vi "TrackAndRotateOmegaCopy.vi"() -> ()   [LabVIEW 2017]
doc: "This example shows how to monitor the measured value and how to set the position while open or closed loop controlled."
uses:
  <vilib>/ULx/Read.llb/ULx Read (Analog 2D DBL NChan NSamp).vi
panel:
  out "i":i32
  in  "Tab Control":enum32{"Page 1", "Page 2", "Page 3"}(tab)
  out "Connected":bool
  out "VISA resource name":refnum<visa-resource-name>="ASRL7::INSTR"
  out "Current position":dbl
  in  "Step size (deg.)":dbl=10.0
  in  "Abort 2":bool
  in  "Nb of steps":i32=50000
  out "Is Ready?":bool
  out "Times":dbl[](array[numeric])
  # "3"
  # "(c) 2012 piezosystem jena GmbH. ALL RIGHTS RESERVED."
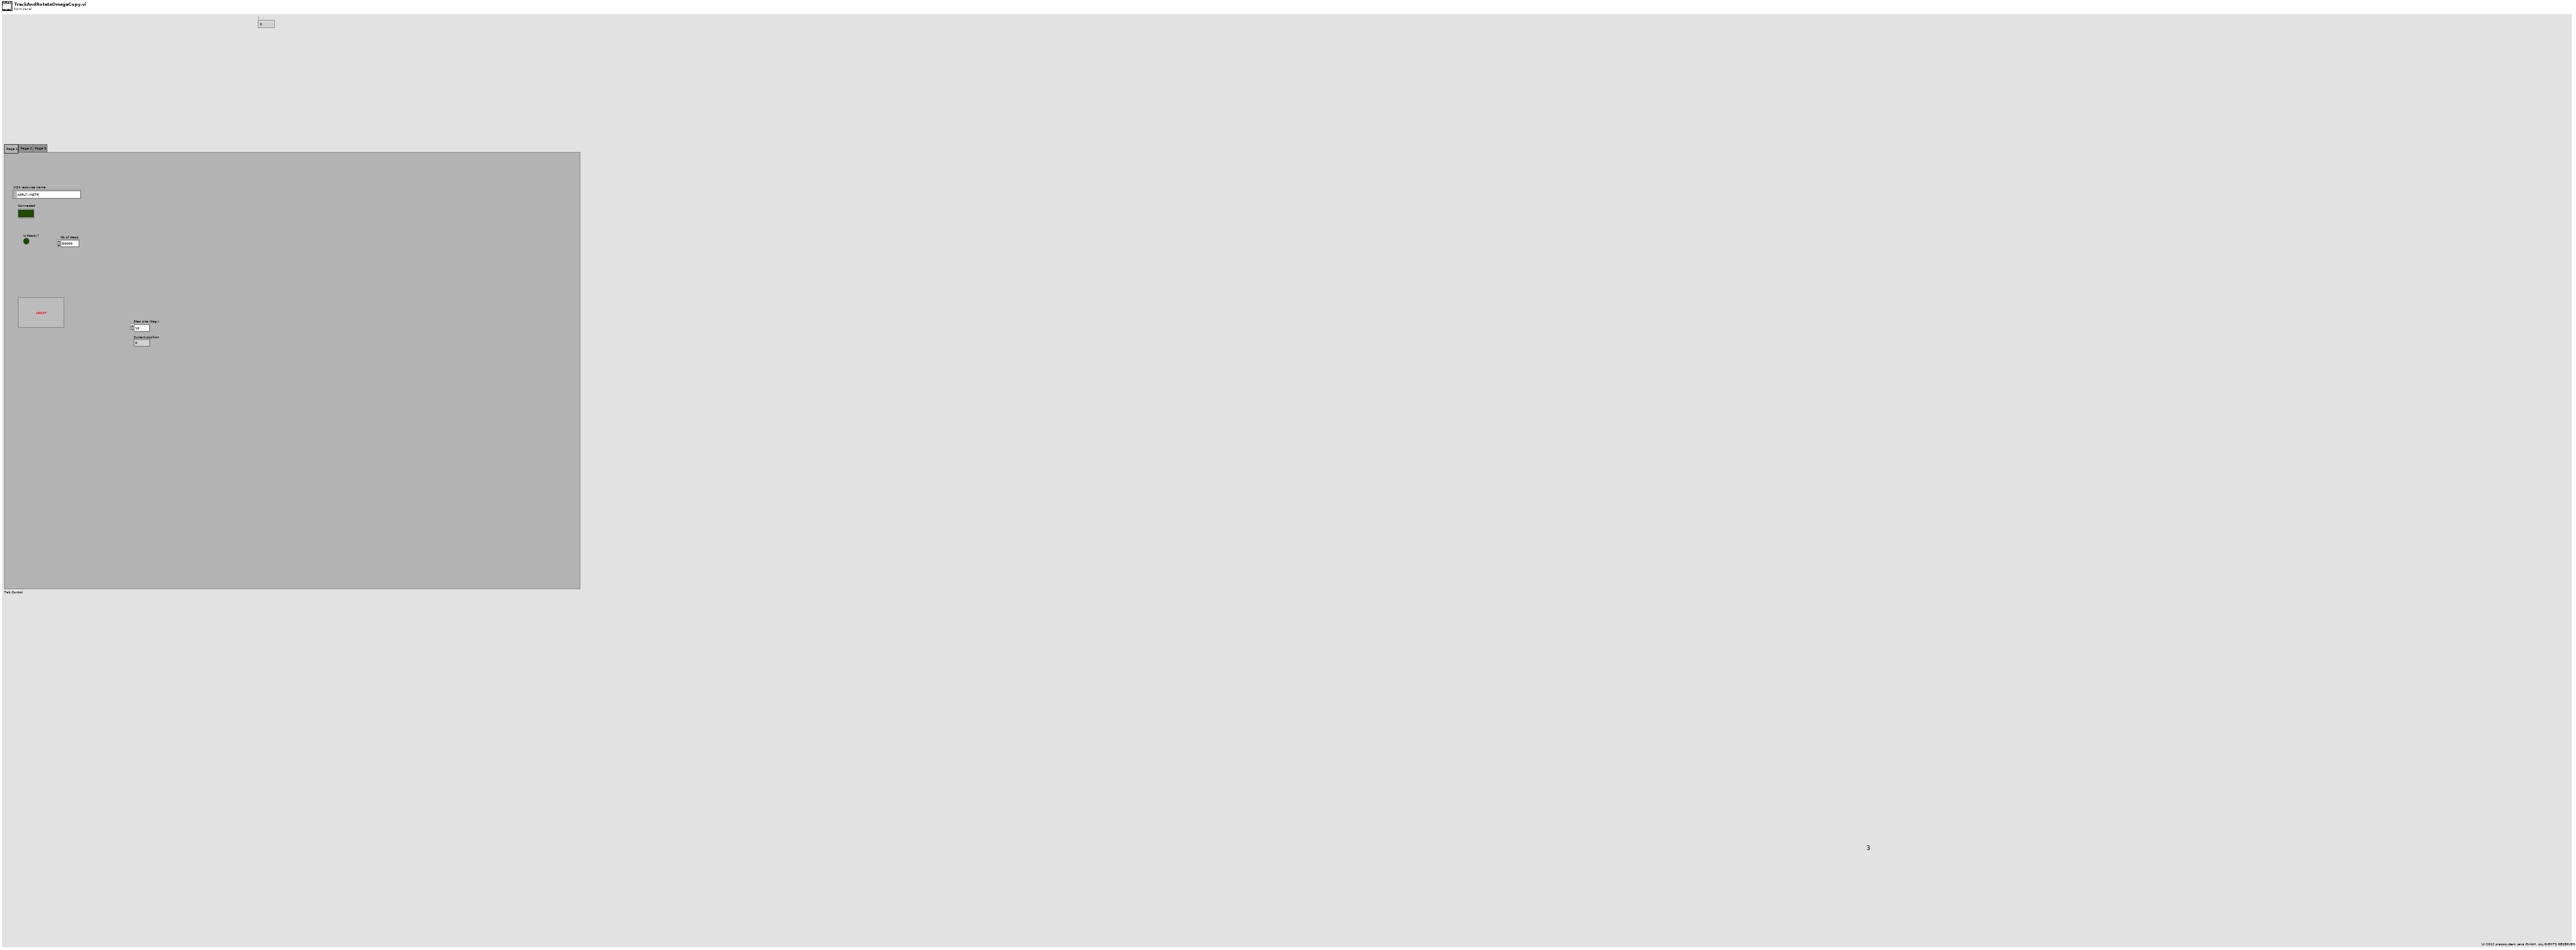
[diagram p1: front panel]
types:
  T1 = cluster{"VISA resource name":refnum<visa-resource-name>, "Device name":string, "Controller address":i32, "error":errorcluster}
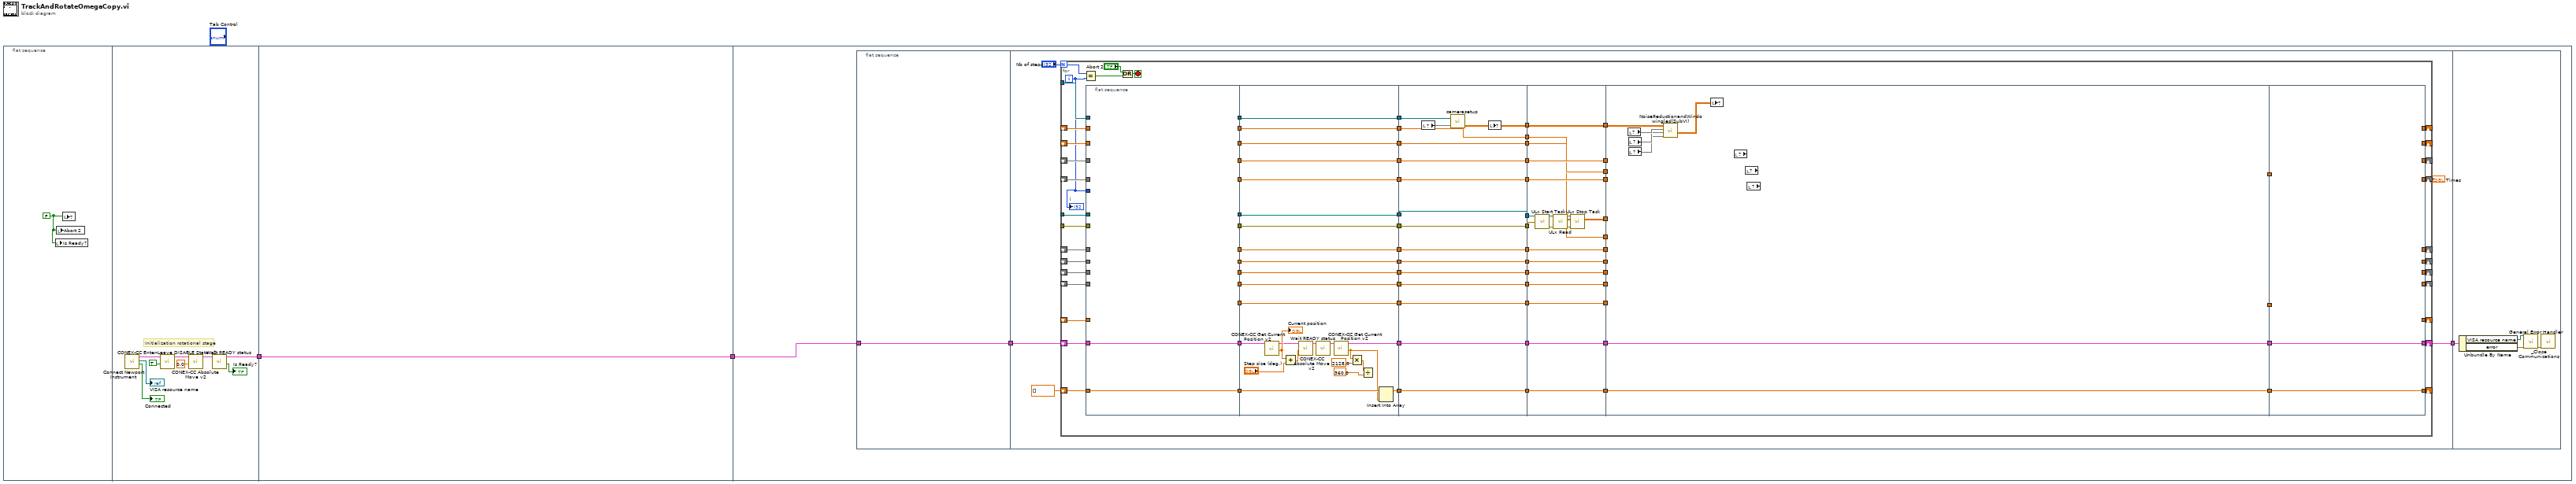
[diagram p0: block diagram]
diagram:
  n1 = flat-sequence {
    tunnel: [w7] -> w1
    tunnel: [w13] -> w2
    tunnel: w1 -> [w13]
    tunnel: w2 -> [w14]
    frame #0 {
      w3 = FALSE
      n2 = local write "Is Ready?"(w3) -> ()
      n3 = local write "Abort 2"(w3) -> ()
      n4 = local write item#-1(w3) -> ()
    }
    frame #1 {
      # "Initialization rotational stage"
      n5 = call <userlib>:"Connect Newport Instrument.vi"() -> ("Connected"=→"Connected":bool, "VISA resource name (duplicate)"=→"VISA resource name":refnum<visa-resource-name>, "Device Connection Cluster"=w10:T1)  [unwired: 7 in, 2 out]
      n6 = call <userlib>:"CONEX-CC Enter-Leave DISABLE State v2.vi"("Ready? (false=DISABLE true=READY)"=TRUE, "Connection Cluster in"=w10) -> ("Connection Cluster out"=w9:T1)  [unwired: 7 in]
      n7 = call <userlib>:"CONEX-CC Absolute Move v2.vi"("Target position"=0.0, "Connection Cluster in"=w9) -> ("Connection Cluster out"=w8:T1)  [unwired: 7 in]
      n8 = call <userlib>:"Wait READY status.vi"("Connection Cluster in"=w8) -> ("IsReady?"=→"Is Ready?":bool, "Connection Cluster out"=w7:T1)  [unwired: 9 in]
    }
    frame #2 {
    }
    frame #3 {
      n9 = flat-sequence {
        tunnel: [w17] -> w16
        tunnel: w14 -> [w17]
        tunnel: w16 -> [w22]
        tunnel: [w21] -> w15
        tunnel: w15 -> [w196]
        frame #0 {
        }
        frame #1 {
          n10 = for {
            N: "Nb of steps" -> [w79]
            shift-right: [w100] -> _
            shift-left: _ -> [w112]
            tunnel: _ -> [w111]
            tunnel: _ -> [w110]
            shift-right: [w109] -> _
            shift-left: _ -> [w108]
            shift-right: [w107] -> _
            shift-left: _ -> [w106]
            shift-right: [w104] -> _
            shift-left: _ -> [w105]
            shift-right: [w102] -> _
            shift-left: _ -> [w103]
            tunnel: _ -> [w99]
            shift-right: [w80] -> w19
            shift-left: _ -> [w90]
            shift-right: [w74] -> _
            shift-left: [w78] -> w24
            shift-right: [w70] -> _
            shift-left: [w73] -> w23
            shift-right: [w66] -> w21
            shift-left: w22 -> [w65]
            shift-right: [w34] -> _
            shift-left: dbl[] [] -> [w40]
            shift-right: [w26] -> _
            shift-left: [w32] -> w18
            i -> [w33]
            stop <- w114 stop-if-true
            n11 = Equal?(x=w79, y=w33) -> (x = y?=w101:bool)
            n12 = flat-sequence {
              tunnel: w99 -> [_]
              tunnel: w112 -> [_]
              tunnel: w111 -> [_]
              tunnel: w110 -> [_]
              tunnel: w108 -> [_]
              tunnel: w106 -> [_]
              tunnel: w105 -> [_]
              tunnel: w103 -> [_]
              tunnel: [_] -> w64
              tunnel: [_] -> w62
              tunnel: [_] -> w60
              tunnel: [_] -> w58
              tunnel: [_] -> w56
              tunnel: [_] -> w54
              tunnel: [_] -> w52
              tunnel: [_] -> w50
              tunnel: w90 -> [_]
              tunnel: [_] -> w48
              tunnel: w33 -> [_]
              tunnel: [_] -> w46
              tunnel: w78 -> [_]
              tunnel: [_] -> w44
              tunnel: w73 -> [_]
              tunnel: w65 -> [w117]
              tunnel: [w117] -> w41
              tunnel: w40 -> [w116]
              tunnel: [w116] -> w39
              tunnel: w32 -> [w115]
              tunnel: [_] -> w31
              tunnel: w64 -> [w143]
              tunnel: [w143] -> w63
              tunnel: w62 -> [w142]
              tunnel: [w142] -> w61
              tunnel: w60 -> [w141]
              tunnel: [w141] -> w59
              tunnel: w58 -> [w140]
              tunnel: [w140] -> w57
              tunnel: w56 -> [w139]
              tunnel: [w139] -> w55
              tunnel: w54 -> [w138]
              tunnel: [w138] -> w53
              tunnel: w52 -> [w137]
              tunnel: [w137] -> w51
              tunnel: w50 -> [w136]
              tunnel: [w136] -> w49
              tunnel: w48 -> [w135]
              tunnel: [w135] -> w47
              tunnel: w46 -> [w134]
              tunnel: [w134] -> w45
              tunnel: w44 -> [w133]
              tunnel: [w133] -> w43
              tunnel: [w122] -> w42
              tunnel: w41 -> [w123]
              tunnel: w39 -> [w121]
              tunnel: [w120] -> w38
              tunnel: w31 -> [w118]
              tunnel: [w118] -> w28
              tunnel: [w159] -> w91
              tunnel: [w152] -> w92
              tunnel: [w158] -> w93
              tunnel: [w157] -> w94
              tunnel: [w156] -> w95
              tunnel: [w155] -> w96
              tunnel: [w154] -> w97
              tunnel: [w150] -> w98
              tunnel: w63 -> [w154]
              tunnel: w61 -> [w155]
              tunnel: w59 -> [w156]
              tunnel: w57 -> [w157]
              tunnel: w55 -> [w158]
              tunnel: w53 -> [w152]
              tunnel: w51 -> [w159]
              tunnel: w49 -> [w151]
              tunnel: w47 -> [w149]
              tunnel: [w149] -> w89
              tunnel: w45 -> [w148]
              tunnel: [w148] -> w77
              tunnel: w43 -> [w147]
              tunnel: [w147] -> w72
              tunnel: [w146] -> w67
              tunnel: w42 -> [w146]
              tunnel: w38 -> [w145]
              tunnel: [w145] -> w35
              tunnel: [w144] -> w29
              tunnel: w28 -> [w144]
              tunnel: w98 -> [w178]
              tunnel: [w178] -> w88
              tunnel: w97 -> [w177]
              tunnel: [w177] -> w87
              tunnel: w96 -> [w176]
              tunnel: [w176] -> w86
              tunnel: w95 -> [w175]
              tunnel: [w175] -> w85
              tunnel: w94 -> [w174]
              tunnel: [w174] -> w84
              tunnel: w93 -> [w167]
              tunnel: w92 -> [w168]
              tunnel: w91 -> [w173]
              tunnel: [w173] -> w83
              tunnel: [w166] -> w82
              tunnel: w89 -> [w165]
              tunnel: [w165] -> w81
              tunnel: w77 -> [w164]
              tunnel: [w164] -> w76
              tunnel: w72 -> [w163]
              tunnel: [w163] -> w71
              tunnel: [w162] -> w68
              tunnel: w67 -> [w162]
              tunnel: [w161] -> w36
              tunnel: w35 -> [w161]
              tunnel: [w160] -> w30
              tunnel: w29 -> [w160]
              tunnel: w88 -> [w191]
              tunnel: w87 -> [_]
              tunnel: w86 -> [_]
              tunnel: w85 -> [_]
              tunnel: w84 -> [_]
              tunnel: w83 -> [w189]
              tunnel: w82 -> [_]
              tunnel: w81 -> [w184]
              tunnel: w76 -> [w183]
              tunnel: [_] -> w75
              tunnel: w71 -> [w182]
              tunnel: [w181] -> w69
              tunnel: w68 -> [w181]
              tunnel: [w180] -> w37
              tunnel: w36 -> [w180]
              tunnel: w30 -> [w179]
              tunnel: [_] -> w27
              tunnel: [_] -> w109
              tunnel: [_] -> w107
              tunnel: [_] -> w104
              tunnel: [_] -> w102
              tunnel: [_] -> w100
              tunnel: [_] -> w80
              tunnel: w75 -> [w195]
              tunnel: [_] -> w74
              tunnel: [_] -> w70
              tunnel: w69 -> [w194]
              tunnel: [w194] -> w66
              tunnel: w37 -> [w193]
              tunnel: [w193] -> w34
              tunnel: w27 -> [w192]
              tunnel: [_] -> w26
              frame #0 {
              }
              frame #1 {
                n13 = call <userlib>:"CONEX-CC Get Current Position v2.vi"("Connection Cluster in"=w123) -> ("Current position"=w128:dbl, "Connection Cluster out"=w127:T1)  [unwired: 8 in, 1 out]
                "Current position" <- w128
                n14 = Add(x=w128, y="Step size (deg.)") -> (x+y=w130:dbl)
                n15 = call <userlib>:"CONEX-CC Absolute Move v2.vi"("Target position"=w130, "Connection Cluster in"=w127) -> ("Connection Cluster out"=w126:T1)  [unwired: 7 in]
                n16 = call <userlib>:"Wait READY status.vi"("Connection Cluster in"=w126) -> ("Connection Cluster out"=w131:T1)  [unwired: 9 in, 1 out]
                n17 = call <userlib>:"CONEX-CC Get Current Position v2.vi"("Connection Cluster in"=w131) -> ("Current position"=w119:dbl, "Connection Cluster out"=w122:T1)  [unwired: 8 in, 1 out]
                n18 = Multiply(x=w119, y=2128.0) -> (x*y=w132:dbl)
                n19 = Divide(x=w132, y=360.0) -> ()  [unwired: 1 out]
                n20 = Insert Into Array(array=w121, new element=w119) -> (w120:dbl[])  [unwired: 1 in]
              }
              frame #2 {
                n21 = local read item#-1() -> (w153)
                n22 = call "camerasetup.vi"("Set Exposure"=w153, "Automation Refnum in"=w151) -> ("Original Image"=w150:dbl[][])  [unwired: 1 out]
                n23 = local write item#-1(w150) -> ()
              }
              frame #3 {
                n24 = call <vilib>:"ULx Start Task.vi"("task in"=w168, "error in"=w167) -> ("task out"=w172:refnum<k24>, "error out"=w171:errorcluster)  [unwired: 12 in]
                n25 = call-poly <vilib>:"ULx Read.vi"("task in"=w172, "error in"=w171) -> ("task out"=w170:refnum<k24>, "data"=w166:dbl[][], "error out"=w169:errorcluster)  [unwired: 11 in]
                n26 = call <vilib>:"ULx Stop Task.vi"("error in"=w169, "task in"=w170) -> ()  [unwired: 8 in, 2 out]
              }
              frame #4 {
                n27 = local read item#-1() -> (w190)
                n28 = local read item#-1() -> (w188)
                n29 = local read item#-1() -> (w187)
                n30 = call "NoiseReductionandWindowingled(SubVI).vi"("Cursor.Cursor Y"=w187, "Cursor.Cursor X"=w188, "Window size"=w190, "Original image"=w191) -> ("Windowed image"=w185:dbl[][])  [unwired: 1 in, 2 out]
                n31 = local write item#-1(w185) -> ()
                n32 = local read item#-1() -> (w186)
                n33 = local read item#-1() -> ()  [unwired: 1 out]
                n34 = local read item#-1() -> ()  [unwired: 1 out]
              }
              frame #5 {
              }
            }
            n35 = Or(x="Abort 2", y=w101) -> (x .or. y?=w114:bool)
            "i" <- w33
          }
          "Times" <- w19
        }
        frame #2 {
          n36 = Unbundle By Name(w196) -> ("VISA resource name"=w197:refnum<visa-resource-name>, "error"=w198:errorcluster)
          n37 = call <userlib>:"_Close Communications.vi"("Instrument Channel"=w197, "error in (no error)"=w198) -> ("error out"=w199:errorcluster)  [unwired: 13 in]
          n38 = call <vilib>:"General Error Handler.vi"("error in (no error)"=w199) -> ()  [unwired: 10 in, 5 out]
        }
      }
    }
  }
